vi "push_string_array.vi"(8 "error in (no error)":errorcluster, 10 "value":string[](array[string]), 11 "Lua in":refnum<class "Lua.lvclass">) -> (0 "error out":errorcluster, 3 "Lua out":refnum<class "Lua.lvclass">)   [LabVIEW 2020, in "Lua for LabVIEW.lvlib" / "Lua.lvclass"]
doc: "Push a numeric array to the Lua stack (creates a lua table)."
uses:
  Lua.lvclass
  Lua.lvclass/Lua.ctl
  lib/lua.dll/lua.dll.lvlib
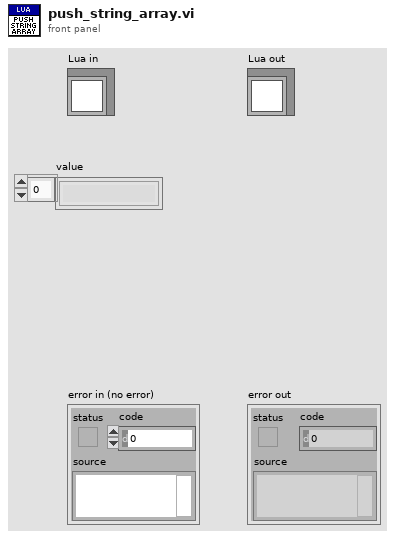
[diagram p1: front panel]
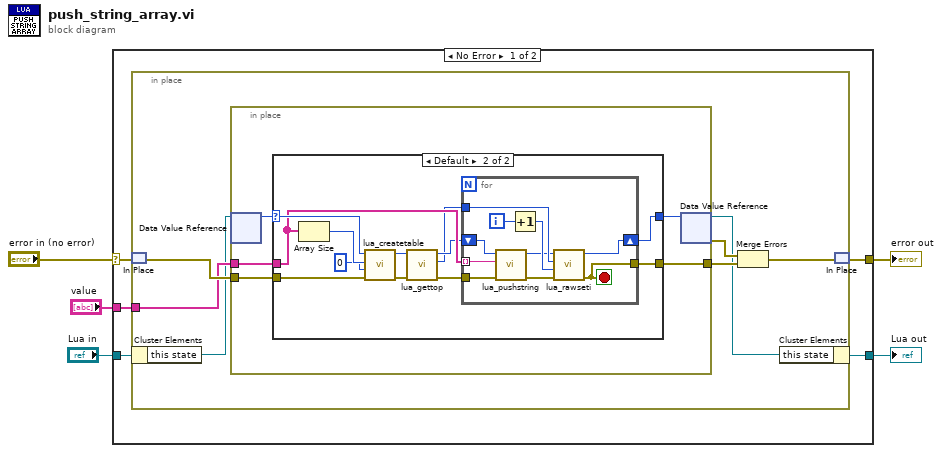
[diagram p0: block diagram]
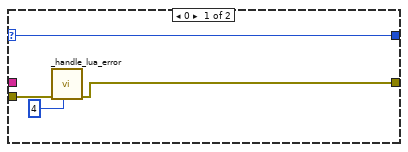
[diagram p2: hidden frame]
diagram:
  n1 = case shown="No Error" "error in (no error)" {
    selector: "error in (no error)" -> [w7 w50]
    tunnel: [w8 w50] -> w4
    tunnel: [w9 w49] -> w2
    tunnel: "Lua in" -> [w10 w49]
    tunnel: "value" -> [w6 _]
    frame No Error {
      n2 = in-place {
        in-place-border: w6 -> [w16]
        n3 = in-place-match #1(w7) -> (w17:errorcluster)
        n4 = in-place-cluster #2(w10) -> ("this state"=w15:refnum<data-value>)
        n5 = in-place {
          in-place-border: w17 -> [w22]
          in-place-border: w16 -> [w21]
          in-place-border: [w18] -> w13
          n6 = in-place-dvr #3(w15) -> (w20:u64)  [unwired: 1 out]
          n7 = case shown="Default" w20 {
            selector: w20 -> [w26 w38]
            tunnel: [w26 w28] -> w19
            tunnel: w22 -> [w23 w36]
            tunnel: [w24 w33] -> w18
            tunnel: w21 -> [_ w34]
            frame 0 {
              n8 = call "_handle_lua_error.vi"("lua status"=4 ("lua_load errcode"), "error in (no error)"=w23) -> ("error out"=w24:errorcluster)  [unwired: 9 in]
            }
            frame Default {
              n9 = Array Size(array=w34) -> (size(s)=w37:i32)
              n10 = call "lua_createtable.vi"("error in (no error)"=w36, "nrec"=0, "narr"=w37, "lua_state_p"=w38) -> ("error out"=w32:errorcluster, "lua_state_p out"=w31:u64)  [unwired: 6 in]
              n11 = call "lua_gettop.vi"("error in (no error)"=w32, "lua_state_p"=w31) -> ("error out"=w30:errorcluster, "index"=w27:i32, "lua_state_p out"=w29:u64)  [unwired: 7 in]
              n12 = for {
                shift-right: [w42] -> w28
                shift-left: w29 -> [w46]
                tunnel: w30 -> [w45]
                tunnel: w34 -> [w48] mode=indexing
                tunnel: [w43] -> w33
                tunnel: w27 -> [w41]
                i -> [w47]
                stop <- w43 stop-if-true
                n13 = call "lua_pushstring.vi"("error in (no error)"=w45, "String"=w48, "lua_state_p"=w46) -> ("error out"=w39:errorcluster, "lua_state_p out"=w40:u64)  [unwired: 7 in]
                n14 = Increment(x=w47) -> (x+1=w44:i32)
                n15 = call "lua_rawseti.vi"("error in (no error)"=w39, "n"=w44, "index"=w41, "lua_state_p"=w40) -> ("error out"=w43:errorcluster, "lua_state_p out"=w42:u64)  [unwired: 6 in]
              }
            }
          }
          n16 = in-place-dvr #3(w19) -> (w11:refnum<data-value>, w14:errorcluster)
        }
        n17 = Merge Errors(w14, w13) -> (w12:errorcluster)
        n18 = in-place-cluster #2("this state"=w11) -> (w9:refnum<class "Lua.lvclass">)
        n19 = in-place-match #1(w12) -> (w8:errorcluster)
      }
    }
    frame Error {
    }
  }
  "error out" <- w4
  "Lua out" <- w2
